vi "EXO1_DatabaseWrite.vi"(0 "LN2 Level_Dewar 1":dbl, 1 "Xe Level":dbl, 2 "Pressure 3":dbl, 3 "Pressure 2":dbl, 5 "Flow Speed":dbl, 6 "Table Name (The table that you want to save the data into)":string="EXO", 7 "LN2 Level_Dewar 2":dbl, 8 "Pressure 1":dbl, 9 "Temperature 3_Thermocouple":dbl, 10 "Temperature 2_DT":dbl, 11 "Temperature 1_PT":dbl) -> ()   [LabVIEW 2012]
uses:
  <vilib>/addons/database/Connection.llb/DB Tools Open Connec (Path).vi
  <vilib>/addons/database/NI_Database_API.lvlib
panel:
  out "current time":timestamp
  in  "stop":bool
  # "EXO DatabaseWrite Sub-VI (I)"
  # "Data List\nTemperature: PT, DT, Thermocouple\nPressure: Sensor1, Sensor2, Sensor3\nLevel Measurement: Xe, Liquid Nitrogen 1, Liquid Nitrogen 2\nFlow Speed: MKS"
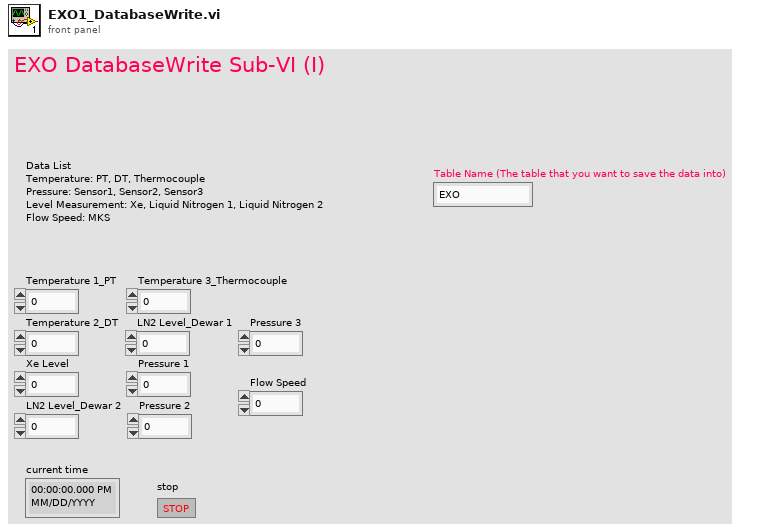
[diagram p1: front panel]
types:
  T1 = typedef "NI_Database_API.lvlib/Conn ObjectReference.ctl" = refnum<k1>
  T2 = cluster{dbl, "date/time string":string, "Temperature 1_PT":dbl, "Temperature 2_DT":dbl, "Temperature 3_Thermocouple":dbl, "Xe Level":dbl, "LN2 Level_Dewar 1":dbl, "LN2 Level_Dewar 2":dbl, "Pressure 1":dbl, "Pressure 2":dbl, "Pressure 3":dbl, "Flow Speed":dbl}
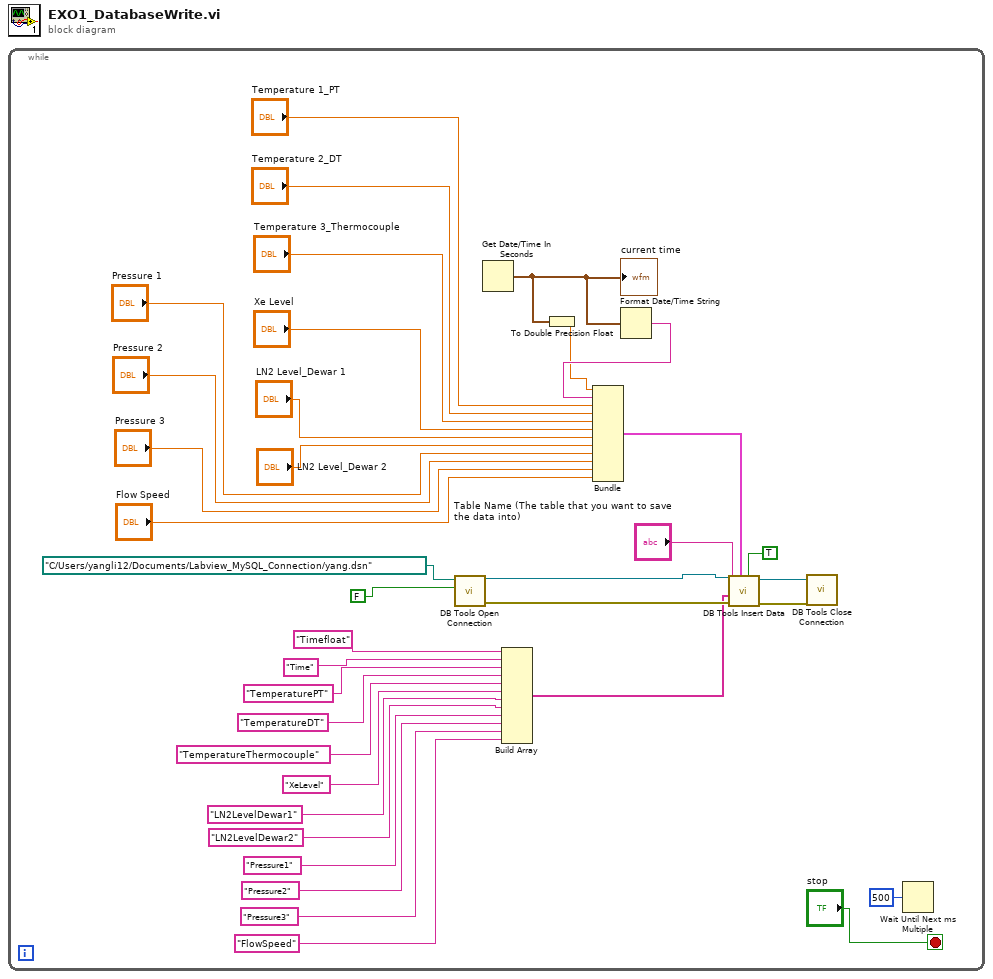
[diagram p0: block diagram]
diagram:
  n1 = while {
    stop <- "stop" stop-if-true
    n2 = call-poly <vilib>:"DB Tools Open Connection.vi"("prompt? (F)"=FALSE, "connection information"=path "C:/Users/yangli12/Documents/Labview_MySQL_Connection/yang.dsn") -> ("error out"=w31:errorcluster, "connection reference"=w32:T1)  [unwired: 6 in]
    n3 = Get Date/Time In Seconds() -> (seconds since 1Jan1904=w23:timestamp)
    "current time" <- w23
    n4 = Build Array("Timefloat" ("element"), "Time" ("table"), "TemperaturePT" ("table"), "TemperatureDT" ("table"), "TemperatureThermocouple" ("table"), "XeLevel" ("table"), "LN2LevelDewar1" ("table"), "LN2LevelDewar2" ("table"), "Pressure1" ("table"), "Pressure2" ("table"), "Pressure3" ("table"), "FlowSpeed" ("table")) -> (w26:string[])
    n5 = To Double Precision Float(number=w23) -> (double precision float=w22:dbl)
    n6 = Format Date/Time String(seconds (now)=w23) -> (date/time string=w24:string)  [unwired: 2 in]
    n7 = Bundle(w22, "date/time string"=w24, "Temperature 1_PT"="Temperature 1_PT", "Temperature 2_DT"="Temperature 2_DT", "Temperature 3_Thermocouple"="Temperature 3_Thermocouple", "Xe Level"="Xe Level", "LN2 Level_Dewar 1"="LN2 Level_Dewar 1", "LN2 Level_Dewar 2"="LN2 Level_Dewar 2", "Pressure 1"="Pressure 1", "Pressure 2"="Pressure 2", "Pressure 3"="Pressure 3", "Flow Speed"="Flow Speed") -> (w30:T2)  [unwired: 1 in]
    n8 = call <vilib>:"DB Tools Insert Data.vi"("create table? (F)"=TRUE, "data"=w30, "error in (no error)"=w31, "columns"=w26, "table"="Table Name (The table that you want to save the data into)", "connection reference"=w32) -> ("error out"=w20:errorcluster, "connection reference out"=w21:T1)  [unwired: 4 in]
    n9 = call <vilib>:"DB Tools Close Connection.vi"("error in (no error)"=w20, "connection reference"=w21) -> ()  [unwired: 5 in, 1 out]
    n10 = Wait Until Next ms Multiple(millisecond multiple=u32 500) -> ()  [unwired: 1 out]
  }
